vi "Read Multipage ImageJ TIFF Header.vi"(7 "TIFF Path":path, 11 "Error":errorcluster) -> (4 "TIF Ref":refnum<file>, 8 "Image Info":T1, 15 "Error":errorcluster)   [LabVIEW 2016]
uses:
  TIF Read Image Information.ctl
panel:
  out "string":string
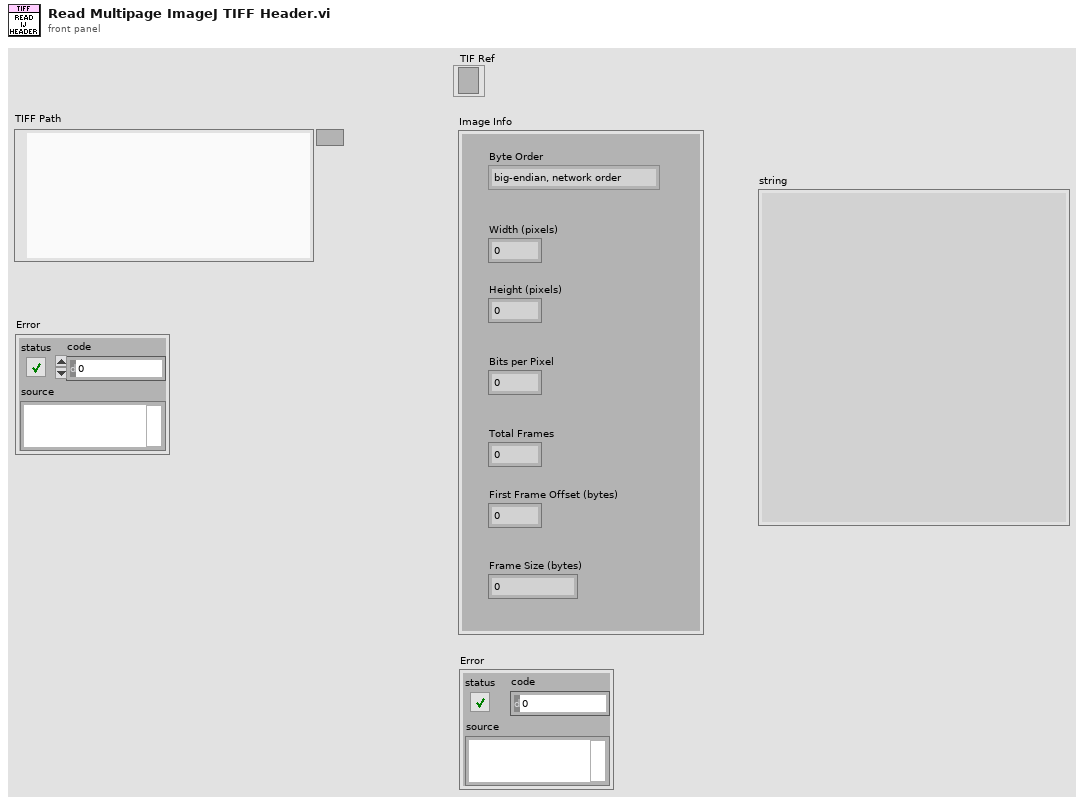
[diagram p1: front panel]
types:
  T1 = typedef "TIF Read Image Information.ctl" = cluster{"Byte Order":enum16{"big-endian, network order", "native, host order", "little-endian"}, "Width (pixels)":i32, "Height (pixels)":i32, "Bits per Pixel":u8, "Total Frames":u32, "First Frame Offset (bytes)":u32, "Frame Size (bytes)":u32}
  T2 = enum16{"big-endian, network order", "native, host order", "little-endian"}
  T3 = enum16{"open", "replace", "create", "open or create", "replace or create", "replace or create with confirmation"}
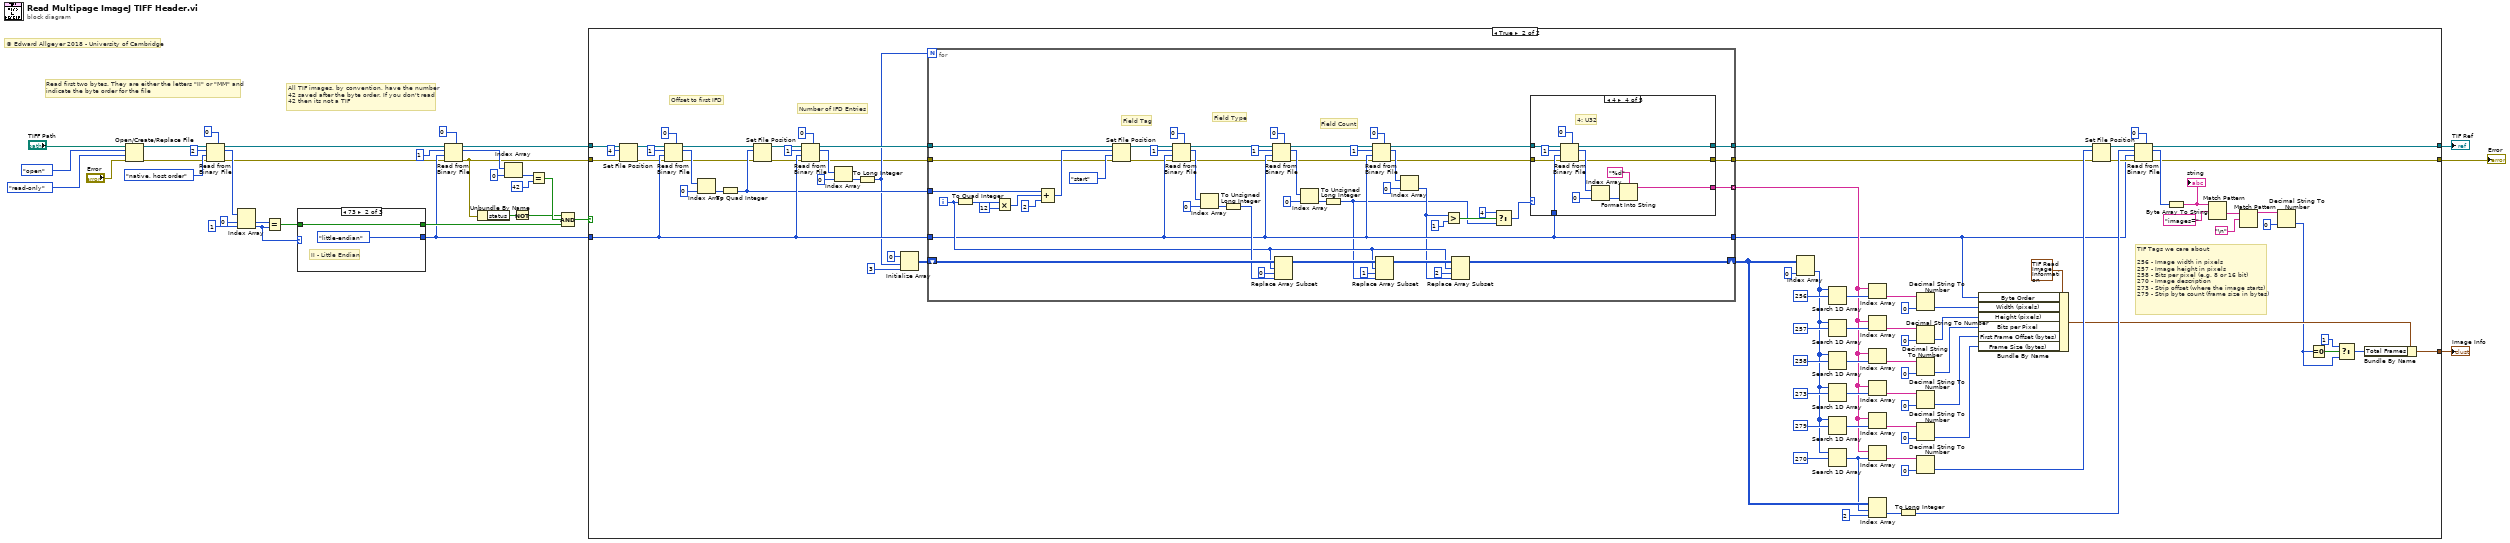
[diagram p0: block diagram]
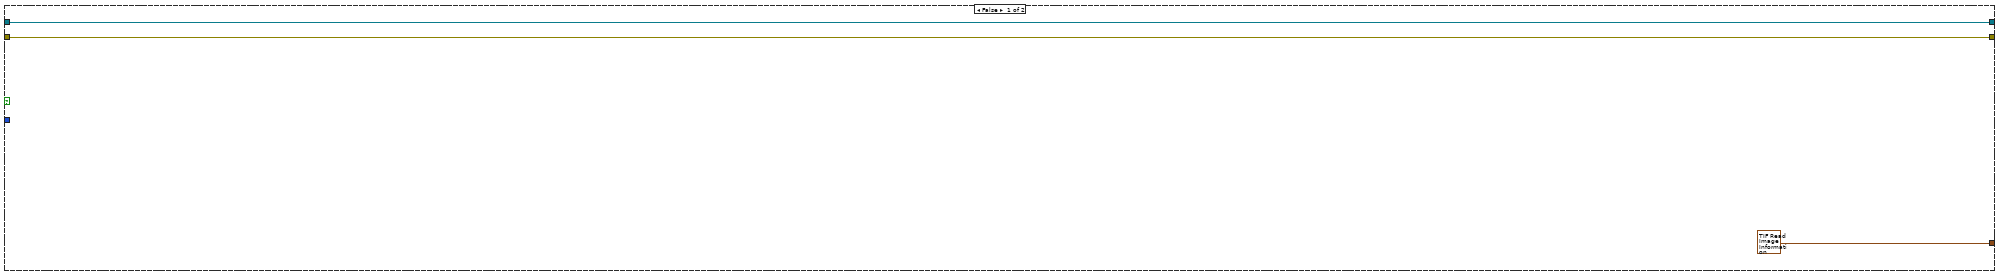
[diagram p2: hidden frame]
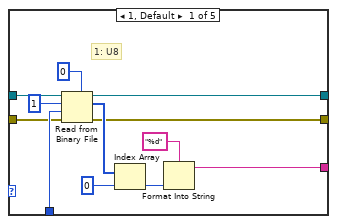
[diagram p3: hidden frame]
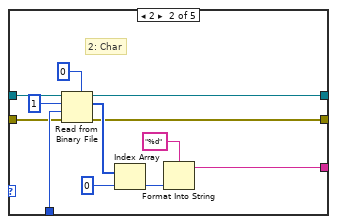
[diagram p4: hidden frame]
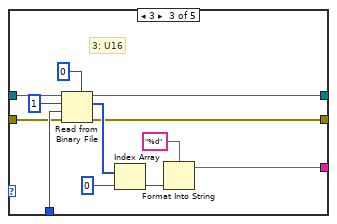
[diagram p5: hidden frame]
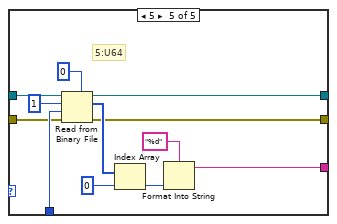
[diagram p6: hidden frame]
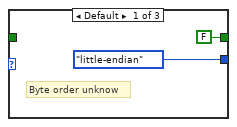
[diagram p7: hidden frame]
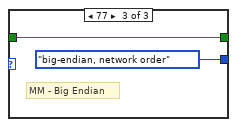
[diagram p8: hidden frame]
diagram:
  # "© Edward Allgeyer 2018 - University of Cambridge"
  # "All TIF images, by convention, have the number\n42 saved after the byte order. If you don't read\n42 then its not a TIF"
  # "Read first two bytes. They are either the letters \"II\" or \"MM\" and\nindicate the byte order for the file"
  n1 = Open/Create/Replace File(file path (use dialog)="TIFF Path", error in="Error", operation (0:open)=T3."open", access (0:read/write)=enum16{"read/write", "read-only", "write-only"}."read-only") -> (refnum out=w31:refnum<file>, error out=w9:errorcluster)  [unwired: 2 in, 1 out]
  n2 = Read from Binary File(5:u8 0, 8:w9, 9:T2."native, host order" ("byte order (0:big-endian, network order)"), 10:2 ("count (1)"), 11:w31) -> (0:w8:errorcluster, 2:w27:u8[], 3:w21:refnum<file>)  [unwired: 1 in, 1 out]
  n3 = Index Array(array=w27, index #1=0 ("index"), index #2=1 ("index")) -> (element #1=w24:u8, element #2=w23:u8)
  n4 = Equal?(x=w24, y=w23) -> (x = y?=w22:bool)
  n5 = case shown="73" w23 {
    tunnel: [T2."little-endian" ("byte order (0:big-endian, network order)") T2."little-endian" ("byte order (0:big-endian, network order)") T2."big-endian, network order" ("byte order (0:big-endian, network order)")] -> w11
    tunnel: w22 -> [_ w37 w39]
    tunnel: [FALSE w37 w39] -> w14
    frame Default {
      # "Byte order unknow"
    }
    frame 73 {
      # "II - Little Endian"
    }
    frame 77 {
      # "MM - Big Endian"
    }
  }
  n6 = Read from Binary File(5:u16 0, 8:w8, 9:w11, 10:1 ("count (1)"), 11:w21) -> (0:w5:errorcluster, 2:w18:u16[], 3:w12:refnum<file>)  [unwired: 1 in, 1 out]
  n7 = Unbundle By Name(w5) -> ("status"=w7:bool)
  n8 = Index Array(array=w18, index=0) -> (element=w16:u16)
  n9 = Not(x=w7) -> (.not. x?=w6:bool)
  n10 = Equal?(x=w16, y=u16 42) -> (x = y?=w13:bool)
  n11 = Compound Arithmetic op=AND(w6, w13, w14) -> (w4:bool)
  n12 = case shown="True" w4 {
    tunnel: w12 -> [w42 w129]
    tunnel: w11 -> [_ w128]
    tunnel: [T1 {"Byte Order"=enum."big-endian, network order", "Width (pixels)"=0, "Height (pixels)"=0, "Bits per Pixel"=0, "Total Frames"=0, "First Frame Offset (bytes)"=0, "Frame Size (bytes)"=0} ("Image Information") w44] -> w10
    tunnel: w5 -> [w43 w58]
    tunnel: [w42 w51] -> w3
    tunnel: [w43 w50] -> w2
    frame False {
    }
    frame True {
      # "Number of IFD Entries"
      # "Offset to first IFD"
      # "TIF Tags we care about\n\n256 - Image width in pixels\n257 - Image height in pixels\n258 - Bits per pixel (e.g. 8 or 16 bit)\n270 - Image description\n273 - Strip offset (where the image starts)\n279 - Strip byte count (frame size in bytes)"
      n13 = Set File Position(offset (in bytes) (0)=i64 4, refnum=w129, error in=w58) -> (refnum out=w69:refnum<file>, error out=w57:errorcluster)  [unwired: 1 in]
      n14 = Read from Binary File(5:u32 0, 8:w57, 9:w128, 10:1 ("count (1)"), 11:w69) -> (0:w56:errorcluster, 2:w76:u32[], 3:w68:refnum<file>)  [unwired: 1 in, 1 out]
      n15 = Index Array(array=w76, index=0) -> (element=w67:u32)
      n16 = To Quad Integer(1:w67) -> (0:w63:i64)
      n17 = Set File Position(offset (in bytes) (0)=w63, refnum=w68, error in=w56) -> (refnum out=w66:refnum<file>, error out=w55:errorcluster)  [unwired: 1 in]
      n18 = Read from Binary File(5:u16 0, 8:w55, 9:w128, 10:1 ("count (1)"), 11:w66) -> (0:w54:errorcluster, 2:w73:u16[], 3:w64:refnum<file>)  [unwired: 1 in, 1 out]
      n19 = Index Array(array=w73, index=0) -> (element=w65:u16)
      n20 = To Long Integer(number=w65) -> (32bit integer=w61:i32)
      n21 = Initialize Array(u32 0 ("element"), w61, 3 ("dimension size")) -> (w59:u32[][])
      n22 = for {
        N: w61 -> [_]
        tunnel: w64 -> [w179]
        tunnel: w128 -> [w142]
        tunnel: w63 -> [w176]
        tunnel: [w144] -> w92
        shift-right: [w146] -> w95
        shift-left: w59 -> [w154]
        tunnel: [w143] -> w114 mode=indexing
        tunnel: [w142] -> w49
        tunnel: w54 -> [w141]
        tunnel: [w136] -> w53
        i -> [w147]
        # "Field Count"
        # "Field Type"
        # "Field Tag"
        n23 = To Quad Integer(1:w147) -> (0:w178:i64)
        n24 = Multiply(x=w178, y=i64 12) -> (x*y=w175:i64)
        n25 = Compound Arithmetic op=ADD(w176, w175, i64 2 ("y")) -> (w172:i64)
        n26 = Set File Position(offset (in bytes) (0)=w172, refnum=w179, from (0:start)=enum16{"start", "end", "current"}."start", error in=w141) -> (refnum out=w173:refnum<file>, error out=w140:errorcluster)
        n27 = Read from Binary File(5:u16 0, 8:w140, 9:w142, 10:1 ("count (1)"), 11:w173) -> (0:w139:errorcluster, 2:w168:u16[], 3:w162:refnum<file>)  [unwired: 1 in, 1 out]
        n28 = Index Array(array=w168, index=0) -> (element=w156:u16)
        n29 = To Unsigned Long Integer(number=w156) -> (unsigned 32bit integer=w152:u32)
        n30 = Read from Binary File(5:u16 0, 8:w139, 9:w142, 10:1 ("count (1)"), 11:w162) -> (0:w138:errorcluster, 2:w165:u16[], 3:w157:refnum<file>)  [unwired: 1 in, 1 out]
        n31 = Replace Array Subset(array=w154, new element=w152, index (row)=w147, index (col)=0 ("disabled index (col)")) -> (w151:u32[][])
        n32 = Index Array(array=w165, index=0) -> (element=w155:u16)
        n33 = To Unsigned Long Integer(number=w155) -> (unsigned 32bit integer=w132:u32)
        n34 = Read from Binary File(5:u32 0, 8:w138, 9:w142, 10:1 ("count (1)"), 11:w157) -> (0:w137:errorcluster, 2:w159:u32[], 3:w145:refnum<file>)  [unwired: 1 in, 1 out]
        n35 = Replace Array Subset(array=w151, new element=w132, index (row)=w147, index (col)=1 ("disabled index (col)")) -> (w149:u32[][])
        n36 = Index Array(array=w159, index=0) -> (element=w135:u32)
        n37 = Greater?(x=w135, y=u32 1) -> (0:w133:bool)
        n38 = Replace Array Subset(array=w149, new element=w135, index (row)=w147, index (col)=2 ("disabled index (col)")) -> (w146:u32[][])
        n39 = Select(t=u32 4, s=w133, f=w132) -> (s? t:f=w131:u32)
        n40 = case shown="4" w131 {
          tunnel: w145 -> [w191 w203 w215 w227 w239]
          tunnel: [w189 w201 w213 w225 w237] -> w144
          tunnel: w142 -> [w188 w200 w212 w224 w236]
          tunnel: [w182 w194 w206 w218 w230] -> w143
          tunnel: w137 -> [w181 w193 w205 w217 w229]
          tunnel: [w180 w192 w204 w216 w228] -> w136
          frame 1, Default {
            # "1: U8"
            n41 = Read from Binary File(5:u8 0 ("index"), 8:w181, 9:w188, 10:1 ("count (1)"), 11:w191) -> (0:w180:errorcluster, 2:w186:u8[], 3:w189:refnum<file>)  [unwired: 1 in, 1 out]
            n42 = Index Array(array=w186, index=0) -> (element=w184:u8)
            n43 = Format Into String(format string="%d", w184) -> (resulting string=w182:string)  [unwired: 2 in, 1 out]
          }
          frame 2 {
            # "2: Char"
            n44 = Read from Binary File(5:u8 0 ("index"), 8:w193, 9:w200, 10:1 ("count (1)"), 11:w203) -> (0:w192:errorcluster, 2:w198:u8[], 3:w201:refnum<file>)  [unwired: 1 in, 1 out]
            n45 = Index Array(array=w198, index=0) -> (element=w196:u8)
            n46 = Format Into String(format string="%d", w196) -> (resulting string=w194:string)  [unwired: 2 in, 1 out]
          }
          frame 3 {
            # "3: U16"
            n47 = Read from Binary File(5:u16 0 ("index"), 8:w205, 9:w212, 10:1 ("count (1)"), 11:w215) -> (0:w204:errorcluster, 2:w210:u16[], 3:w213:refnum<file>)  [unwired: 1 in, 1 out]
            n48 = Index Array(array=w210, index=0) -> (element=w208:u16)
            n49 = Format Into String(format string="%d", w208) -> (resulting string=w206:string)  [unwired: 2 in, 1 out]
          }
          frame 4 {
            # "4: U32"
            n50 = Read from Binary File(5:u32 0 ("index"), 8:w217, 9:w224, 10:1 ("count (1)"), 11:w227) -> (0:w216:errorcluster, 2:w222:u32[], 3:w225:refnum<file>)  [unwired: 1 in, 1 out]
            n51 = Index Array(array=w222, index=0) -> (element=w220:u32)
            n52 = Format Into String(format string="%d", w220) -> (resulting string=w218:string)  [unwired: 2 in, 1 out]
          }
          frame 5 {
            # "5:U64"
            n53 = Read from Binary File(5:u32 0 ("index"), 8:w229, 9:w236, 10:1 ("count (1)"), 11:w239) -> (0:w228:errorcluster, 2:w234:u32[], 3:w237:refnum<file>)  [unwired: 1 in, 1 out]
            n54 = Index Array(array=w234, index=0) -> (element=w232:u32)
            n55 = Format Into String(format string="%d", w232) -> (resulting string=w230:string)  [unwired: 2 in, 1 out]
          }
        }
      }
      n56 = Index Array(array=w95, index (col)=0 ("disabled index (col)")) -> (element=w119:u32[])  [unwired: 1 in]
      n57 = Search 1D Array(1D array=w119, element=u32 256) -> (index of element=w124:i32)  [unwired: 1 in]
      n58 = Search 1D Array(1D array=w119, element=u32 257) -> (index of element=w118:i32)  [unwired: 1 in]
      n59 = Search 1D Array(1D array=w119, element=u32 258) -> (index of element=w117:i32)  [unwired: 1 in]
      n60 = Search 1D Array(1D array=w119, element=u32 273) -> (index of element=w116:i32)  [unwired: 1 in]
      n61 = Search 1D Array(1D array=w119, element=u32 279) -> (index of element=w115:i32)  [unwired: 1 in]
      n62 = Search 1D Array(1D array=w119, element=u32 270) -> (index of element=w94:i32)  [unwired: 1 in]
      n63 = Index Array(array=w114, index=w124) -> (element=w112:string)
      n64 = Index Array(array=w114, index=w118) -> (element=w108:string)
      n65 = Index Array(array=w114, index=w117) -> (element=w105:string)
      n66 = Index Array(array=w114, index=w116) -> (element=w102:string)
      n67 = Index Array(array=w114, index=w115) -> (element=w99:string)
      n68 = Index Array(array=w114, index=w94) -> (element=w96:string)
      n69 = Index Array(array=w95, index (row)=w94, index (col)=2 ("disabled index (col)")) -> (element=w89:u32)
      n70 = To Long Integer(number=w89) -> (32bit integer=w88:i32)
      n71 = Decimal String To Number(string=w112, default (0L)=0 ("default (0 I32)")) -> (number=w110:i32)  [unwired: 1 in, 1 out]
      n72 = Decimal String To Number(string=w108, default (0L)=0 ("default (0 I32)")) -> (number=w107:i32)  [unwired: 1 in, 1 out]
      n73 = Decimal String To Number(string=w105, default (0L)=u8 0 ("default (0 I32)")) -> (number=w104:u8)  [unwired: 1 in, 1 out]
      n74 = Decimal String To Number(string=w102, default (0L)=u32 0 ("default (0 I32)")) -> (number=w100:u32)  [unwired: 1 in, 1 out]
      n75 = Decimal String To Number(string=w99, default (0L)=u32 0 ("default (0 I32)")) -> (number=w98:u32)  [unwired: 1 in, 1 out]
      n76 = Decimal String To Number(string=w96, default (0L)=i64 0 ("default (0 I32)")) -> (number=w91:i64)  [unwired: 1 in, 1 out]
      n77 = Bundle By Name(cluster=T1 {"Byte Order"=enum."big-endian, network order", "Width (pixels)"=0, "Height (pixels)"=0, "Bits per Pixel"=0, "Total Frames"=0, "First Frame Offset (bytes)"=0, "Frame Size (bytes)"=0} ("Image Information"), "Byte Order"=w49, "Width (pixels)"=w110, "Height (pixels)"=w107, "Bits per Pixel"=w104, "First Frame Offset (bytes)"=w100, "Frame Size (bytes)"=w98) -> (w79:T1)
      n78 = Set File Position(offset (in bytes) (0)=w91, refnum=w92, error in=w53) -> (refnum out=w90:refnum<file>, error out=w52:errorcluster)  [unwired: 1 in]
      n79 = Read from Binary File(5:u8 0, 8:w52, 9:w49, 10:w88, 11:w90) -> (0:w50:errorcluster, 2:w86:u8[], 3:w51:refnum<file>)  [unwired: 1 in, 1 out]
      n80 = Byte Array To String(unsigned byte array=w86) -> (string=w85:string)
      "string" <- w85
      n81 = Match Pattern(string=w85, regular expression="images=") -> (after substring=w83:string)  [unwired: 1 in, 3 out]
      n82 = Match Pattern(string=w83, regular expression="\n") -> (before substring=w80:string)  [unwired: 1 in, 3 out]
      n83 = Decimal String To Number(string=w80, default (0L)=u32 0 ("default (0 I32)")) -> (number=w47:u32)  [unwired: 1 in, 1 out]
      n84 = Equal To 0?(x=w47) -> (x = 0?=w48:bool)
      n85 = Select(t=u32 1, s=w48, f=w47) -> (s? t:f=w45:u32)
      n86 = Bundle By Name(cluster=w79, "Total Frames"=w45) -> (w44:T1)
    }
  }
  "Image Info" <- w10
  "TIF Ref" <- w3
  "Error" <- w2
